vi "ConvertModBusCommand.vi"(9 "DeviceName":string="LinkName=='Ethernet'", 11 "DB Reference In":i32) -> (3 "Modbus Command":T1[](array[typedef]) {"Function Code" items=["Read Coils"=1, "Read Discrete Inputs"=2, "Read Holding Registers"=3, "Read Input Registers"=4, "Write Single Coil"=5, "Write Single Register"=6, "Read Exception Status"=7, "Write Multiple Coils"=15, "Write Multiple Registers"=16]})   [LabVIEW 2020, in "ModBusCommon.lvlib"]
doc: "组织ModBus指令"
uses:
  ModBusCommon.lvlib
  DriverCommon/MB Modbus Command.ctl
  SQLiteBase.lvlib
  DriverCommon.lvlib
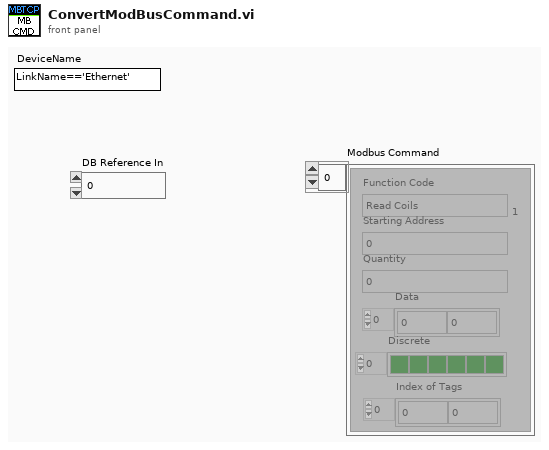
[diagram p1: front panel]
types:
  T1 = typedef "DriverCommon.lvlib/MB Modbus Command.ctl" = cluster{"Function Code":u8, "Starting Address":u16, "Quantity":u16, "Data":u16[], "Discrete":bool[], "Index of Tags":i32[]}
  T2 = cluster{"Function Code":u8, "Starting Address":u16, "Quantity":u16, "Data":u16[], "Discrete":bool[]}
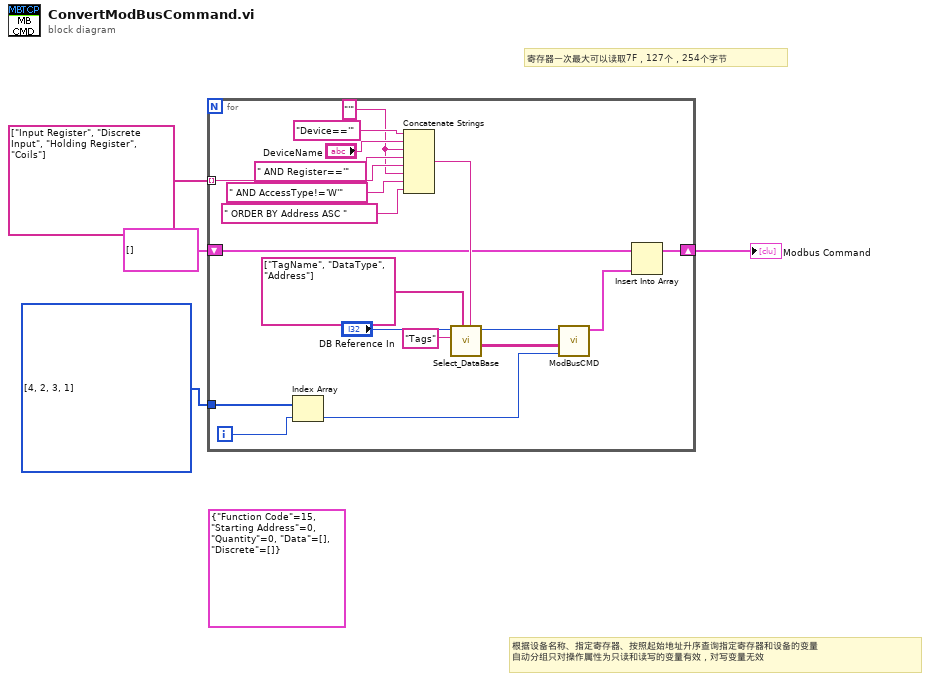
[diagram p0: block diagram]
diagram:
  w3 = u8[] [4, 2, 3, 1] items=["Read Coils"=1, "Read Discrete Inputs"=2, "Read Holding Registers"=3, "Read Input Registers"=4, "Write Single Coil"=5, "Write Single Register"=6, "Read Exception Status"=7, "Write Multiple Coils"=15, "Write Multiple Registers"=16]
  (unwired) T2 {"Function Code"=15, "Starting Address"=0, "Quantity"=0, "Data"=[], "Discrete"=[]} ("Modbus Command")
  # "寄存器一次最大可以读取7F，127个，254个字节"
  # "根据设备名称、指定寄存器、按照起始地址升序查询指定寄存器和设备的变量\n自动分组只对操作属性为只读和读写的变量有效，对写变量无效"
  n1 = for {
    tunnel: string[] ["Input Register", "Discrete Input", "Holding Register", "Coils"] ("Strings []") -> [w16] mode=indexing
    tunnel: w3 -> [w11]
    shift-right: [w8] -> w1
    shift-left: T1[] [] ("ModBus Read Command") -> [w9]
    i -> [w10]
    w15 = "'" ("string")
    n2 = Index Array(array=w11, index=w10) -> (element=w6:u8)
    n3 = Concatenate Strings("Device=='" ("Expression"), "DeviceName", w15, " AND Register=='" ("string"), w16, w15, " AND AccessType!='W'" ("string"), " ORDER BY Address ASC ") -> (w18:string)
    n4 = call "Select_DataBase.vi"("Expression"=w18, "Query Columns"=string[] ["TagName", "DataType", "Address"], "Table name"="Tags", "DB Reference In"="DB Reference In") -> ("Data"=w12:string[][], "DB Reference Out"=w5:i32)  [unwired: 5 in, 1 out]
    n5 = call "ModBusCMD.vi"("Function Code"=w6, "Tag Information"=w12, "DB Reference In"=w5) -> ("ModBus Read Command"=w7:T1[])  [unwired: 8 in]
    n6 = Insert Into Array(array=w9, new element=w7) -> (w8:T1[])  [unwired: 1 in]
  }
  "Modbus Command" <- w1
